vi "Calculate Throughput Metrics.vi"(10 "Channel Count":i32, 11 "Durations":u32[](array[numeric])) -> (2 "Histogram Graph":T2(graph), 3 "Metrics":T1 {"Transfer Rate" format="%.2pB/s"; "Duration Std. Dev." format="%.0f µs"; "Duration Average" format="%.0f µs"})   [LabVIEW 2016]
uses:
  Controls/Throughput Metrics.ctl
  <vilib>/Analysis/NI_AALBase.lvlib
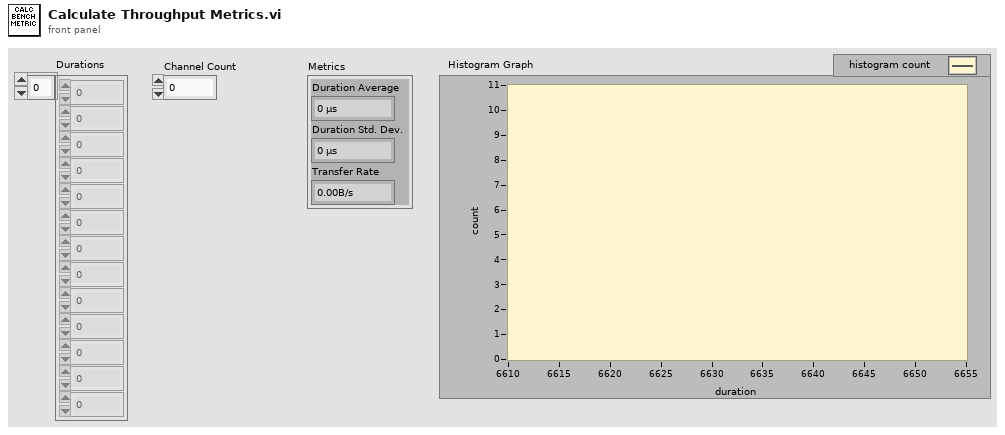
[diagram p1: front panel]
types:
  T1 = typedef "Throughput Metrics.ctl" = cluster{"Duration Average":u32, "Duration Std. Dev.":u32, "Transfer Rate":dbl}
  T2 = cluster{"X Values":dbl[], "Histogram: h(x)":i32[]}
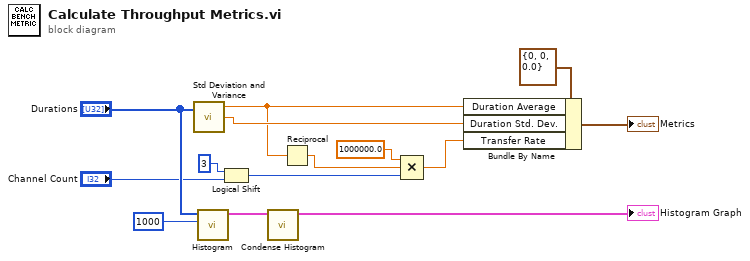
[diagram p0: block diagram]
diagram:
  n1 = call <vilib>:"Std Deviation and Variance.vi"("X"="Durations") -> ("mean"=w7:dbl, "standard deviation"=w11:dbl)  [unwired: 1 in, 1 out]
  n2 = call <vilib>:"Histogram.vi"("intervals"=1000, "X"="Durations") -> ("Histogram Graph"=w2:T2)  [unwired: 6 in, 3 out]
  n3 = Logical Shift(y=i16 3, x="Channel Count") -> (x << y=w8:i32)
  n4 = call "Condense Histogram.vi"("Histogram Graph in"=w2) -> ("Histogram Graph out"=→"Histogram Graph":T2)  [unwired: 10 in]
  n5 = Reciprocal(x=w7) -> (1/x=w6:dbl)
  n6 = Compound Arithmetic op=MULTIPLY(1000000.0 ("value"), w6, w8) -> (w5:dbl)
  n7 = Bundle By Name(cluster=T1 {"Duration Average"=0, "Duration Std. Dev."=0, "Transfer Rate"=0.0} ("Cluster"), "Duration Average"=w7, "Duration Std. Dev."=w11, "Transfer Rate"=w5) -> (→"Metrics":T1)
